vi "run action UI.vi"(8 "error in (no error)":errorcluster, 9 "action display name":string, 10 "action configuration":refnum<class "action configuration.lvclass">, 11 "subpanel state":T1) -> (0 "error out":errorcluster, 3 "subpanel state out":T1)   [LabVIEW 2014, in "Simple Sequencer TBM editor node.lvclass"]
doc: "Opens and runs the VI with the specified action name."
uses:
  Simple Sequencer TBM editor node.lvclass
  sequencer parent classes/action configuration parent/action configuration.lvclass
  subpanel state.ctl
  VI calling template typedef.ctl
  user event typedef.ctl
  action config and UI pairing.ctl
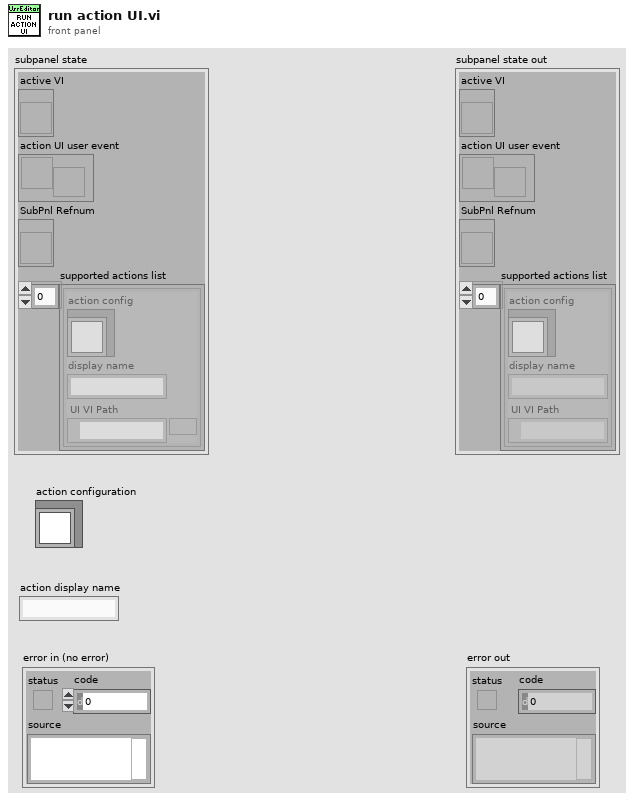
[diagram p1: front panel]
types:
  T1 = typedef "Simple Sequencer TBM editor node.lvclass/subpanel state.ctl" = cluster{"active VI":T2, "action UI user event":refnum<user-event>, "SubPnl Refnum":refnum<vi>, "supported actions list":T3[]}
  T2 = typedef "Simple Sequencer TBM editor node.lvclass/VI calling template typedef.ctl" = refnum<vi>
  T3 = typedef "Simple Sequencer TBM editor node.lvclass/action config and UI pairing.ctl" = cluster{"action config":refnum<class "action configuration.lvclass">, "display name":string, "UI VI Path":path}
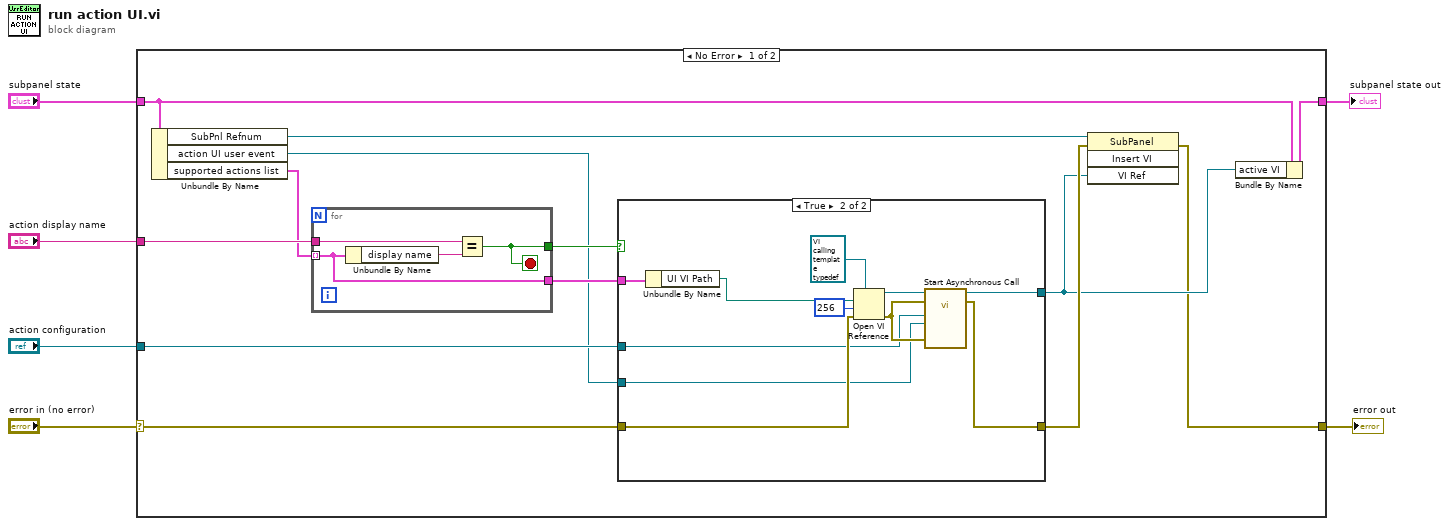
[diagram p0: block diagram]
diagram:
  n1 = case shown="No Error" "error in (no error)" {
    selector: "error in (no error)" -> [w17 w37]
    tunnel: [w8 w37] -> w5
    tunnel: "action display name" -> [w19 _]
    tunnel: "action configuration" -> [w15 _]
    tunnel: "subpanel state" -> [w14 w36]
    tunnel: [w9 w36] -> w1
    frame No Error {
      n2 = Unbundle By Name(w14) -> ("SubPnl Refnum"=w12:refnum<vi>, "action UI user event"=w13:refnum<user-event>, "supported actions list"=w7:T3[])
      n3 = for {
        tunnel: w19 -> [w34]
        tunnel: w7 -> [w32] mode=indexing
        tunnel: [w33] -> w18
        tunnel: [w32] -> w16
        stop <- w33 stop-if-true
        n4 = Unbundle By Name(w32) -> ("display name"=w35:string)
        n5 = Equal?(x=w34, y=w35) -> (x = y?=w33:bool)
      }
      n6 = case shown="True" w18 {
        tunnel: w17 -> [w20 w27]
        tunnel: [w20 w25] -> w11
        tunnel: w16 -> [_ w31]
        tunnel: w15 -> [_ w24]
        tunnel: w13 -> [_ w23]
        tunnel: [_ w22] -> w10
        frame False {
          # "#todo throw not found error"
        }
        frame True {
          n7 = Unbundle By Name(w31) -> ("UI VI Path"=w21:path)
          n8 = Open VI Reference(type specifier VI Refnum (for type only)=T2 refnum, vi path=w21, options=256, error in (no error)=w27) -> (vi reference=w28:T2, error out=w26:errorcluster)  [unwired: 2 in]
          n9 = call-by-ref "Start Asynchronous Call"(reference=w28, error in=w26, 8:"error in (no error)"=w26, "user event"=w23, "action configuration in"=w24) -> (reference out=w22:T2, error out=w25:errorcluster)  [unwired: 7 in, 2 out]
        }
      }
      n10 = invoke on="Invoke Node" class="SubPanel" method="Insert VI"(reference=w12, error in=w11, "VI Ref"=w10) -> (error out=w8:errorcluster)  [unwired: 1 in, 3 out]
      n11 = Bundle By Name(cluster=w14, "active VI"=w10) -> (w9:T1)
    }
    frame Error {
    }
  }
  "error out" <- w5
  "subpanel state out" <- w1
